vi "Lab2_Exercise1_Li_Lim.vi"() -> ()   [LabVIEW 2016]
panel:
  out "String":string
  in  "stop":bool
  out "Waveform Chart":dbl(graph)
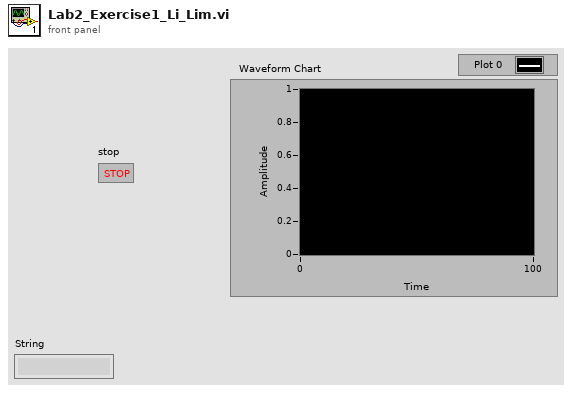
[diagram p1: front panel]
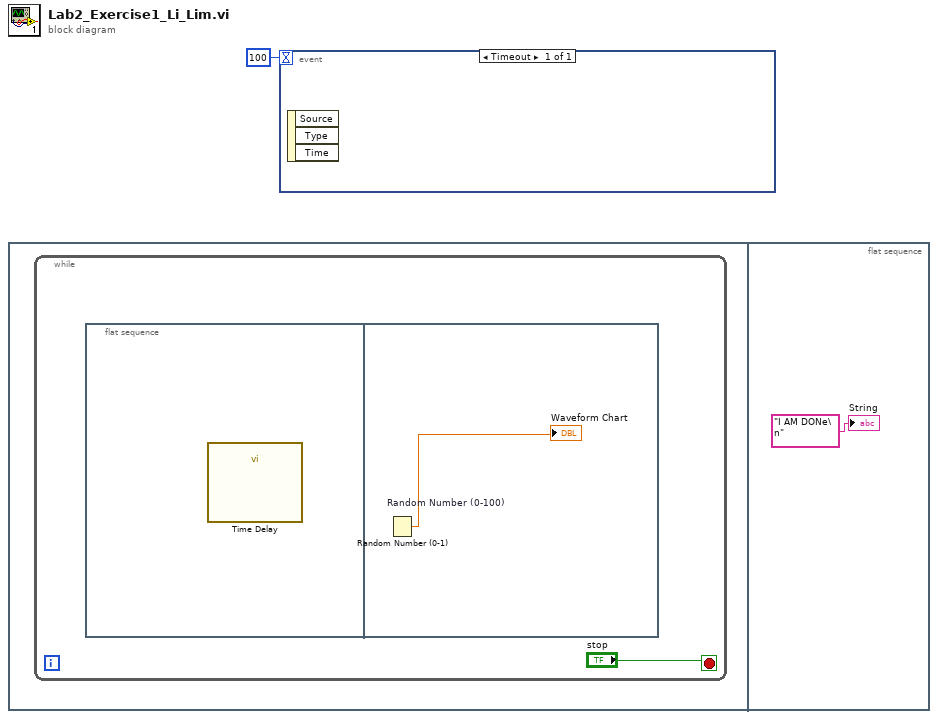
[diagram p0: block diagram]
diagram:
  n1 = flat-sequence {
    frame #0 {
      n2 = while {
        stop <- "stop" stop-if-true
        n3 = flat-sequence {
          frame #0 {
            n4 = call "Time Delay"() -> ()  [unwired: 11 in, 1 out]
          }
          frame #1 {
            n5 = Random Number (0-1) "Random Number (0-100)"() -> (number: 0 to 1=→"Waveform Chart":dbl)
          }
        }
      }
    }
    frame #1 {
      "String" <- "I AM DONe\n" ("String")
    }
  }
  n6 = event shown="[0] Timeout" {
    selector: _ -> [_]
    dyn-events: _ -> [_]
    timeout: 100 -> [_]
    event Timeout {
      n7 = event-data() -> ()  [unwired: 1 in, 3 out]
    }
  }
